vi "Geometric Random.vi"(6 "seed":i32=-1, 7 "reset":bool, 10 "p":dbl=0.5, 11 "samples":i32=128) -> (0 "error":i32, 3 "geometric random data":i32[](array[numeric]))   [LabVIEW 2014, in "NI_Gmath.lvlib"]
doc: "Generates random values from a variate X, where X describes the selected distribution type. You must manually select the polymorphic instance to use."
uses:
  NI_Gmath.lvlib
panel:
  # "Geometric Random"
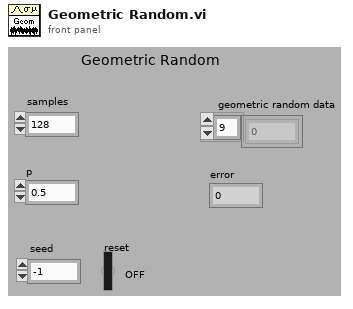
[diagram p1: front panel]
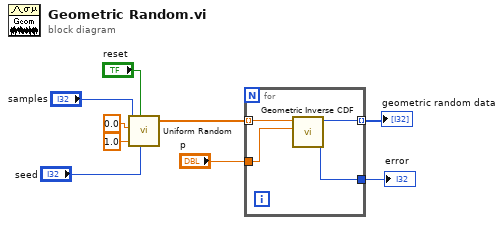
[diagram p0: block diagram]
diagram:
  n1 = call "Uniform Random.vi"("seed"="seed", "reset"="reset", "xmax"=1.0, "xmin"=0.0, "samples"="samples") -> ("uniform random data"=w3:dbl[])  [unwired: 5 in, 1 out]
  n2 = for {
    tunnel: "p" -> [w11]
    tunnel: [w13] -> w9 mode=indexing
    tunnel: [w12] -> w8
    tunnel: w3 -> [w10] mode=indexing
    n3 = call "Geometric Inverse CDF.vi"("p"=w11, "cdf(n)"=w10) -> ("error"=w12:i32, "n"=w13:i32)  [unwired: 8 in]
  }
  "error" <- w8
  "geometric random data" <- w9
